vi "DFD FXP Postprocessing (I16, nCh).vi"(5 "input range":dbl=1.0, 6 "history in":i16[](array[numeric]), 7 "# channels":i32=1, 8 "error in (no error)":errorcluster, 10 "filter":T1={"mSRate_Fs"=1.0, "mSRate_Version"="2.0", "mSRate_Comments"="", "mSRate_OrgCoef"={"type"=enum."Undefined", "gain"=1.0, "coef a (k)"=[], "coef b (v)"=[]}, "mSRate_CurCoef"={"type"=enum."Undefined", "gain"=1.0, "coef a (k)"=[], "coef b (v)"=[]}, "mSRate_Quantized?"=FALSE, "mSRate_QCoef"={"type"=enum."Undefined", "gain"=1.0, "coef a (k)"=[], "coef b (v)"=[]}, "mSRate_QSettings"=[], "mSRate_Order"=0, "mSRate_Scaling"={"mSRate_ScaleByPowerOf2?"=FALSE, "mSRate_ScaleType"=enum."No Norm"}} {"mSRate_QSettings"."source" items=["Coef a/k"=0, "Coef b/v"=7, "Input"=1, "Output"=2, "Multiplicand"=3, "Product"=4, "Sum"=5, "Delay"=6, "Gain"=8]}, 11 "signal in":i16[](array[numeric]) format="%.0x") -> (0 "error out":errorcluster, 3 "signal out":dbl[][](array[numeric]), 4 "history out":i16[](array[numeric]))   [LabVIEW 2017, in "NI_DigFilterLicensed.lvlib"]
doc: "Converts the output signal of a fixed-point filter from a fixed-point integer representation to a floating-point representation. You must manually select the polymorphic instance you want to use."
uses:
  <vilib>/addons/Digital Filter Design/NI_DigFilterLicensed.lvlib
  <vilib>/addons/Digital Filter Design/_Objects.llb/DFD Filter Obj.ctl
  <vilib>/addons/Digital Filter Design/_Objects.llb/DFD Filter Coef.ctl
  <vilib>/addons/Digital Filter Design/_Objects.llb/DFD Filter Structure Type Selector.ctl
  <vilib>/addons/Digital Filter Design/_Objects.llb/dfd_Internal Quantization Settings.ctl
  <vilib>/addons/Digital Filter Design/_Objects.llb/dfd_Internal Quantization Srcs.ctl
  <vilib>/addons/Digital Filter Design/_Objects.llb/DFD Coef Norm Type.ctl
  <vilib>/addons/Digital Filter Design/NI_DigFilter_FXP.lvlib
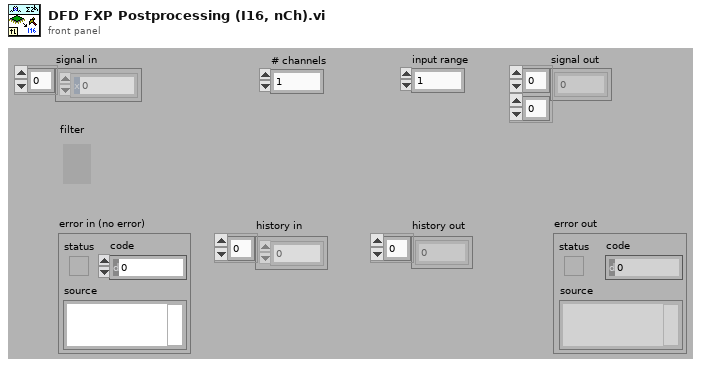
[diagram p1: front panel]
types:
  T1 = typedef "NI_DigFilterLicensed.lvlib/DFD Filter Obj.ctl" = cluster{"mSRate_Fs":dbl, "mSRate_Version":string, "mSRate_Comments":string, "mSRate_OrgCoef":T2, "mSRate_CurCoef":T2, "mSRate_Quantized?":bool, "mSRate_QCoef":T2, "mSRate_QSettings":T4[], "mSRate_Order":i32, "mSRate_Scaling":cluster{"mSRate_ScaleByPowerOf2?":bool, "mSRate_ScaleType":T6}}
  T2 = typedef "NI_DigFilterLicensed.lvlib/DFD Filter Coef.ctl" = cluster{"type":T3, "gain":dbl, "coef a (k)":dbl[], "coef b (v)":dbl[]}
  T3 = typedef "NI_DigFilterLicensed.lvlib/DFD Filter Structure Type Selector.ctl" = enum16{"Undefined", "FIR Direct Form", "FIR Direct Form Transposed", "FIR Symmetric", "FIR Antisymmetric", "IIR Direct Form I", "IIR Direct Form I Transposed", "IIR Direct Form II", "IIR Direct Form II Transposed", "IIR Cascaded Second Order Sections Form I", "IIR Cascaded Second Order Sections Form I Transposed", "IIR Cascaded Second Order Sections Form II", "IIR Cascaded Second Order Sections Form II Transposed", "Lattice Allpass (basic sections)", "Lattice Allpass (one multiplier sections)", "Lattice Allpass (normalized sections)", "Lattice AR (basic sections)", "Lattice AR (one multiplier sections)", "Lattice AR (normalized sections)", "Lattice MA (minimum phase)", "Lattice MA (maximum phase)", "Lattice ARMA (basic sections)", "Lattice ARMA (one multiplier sections)", "Lattice ARMA (normalized sections)"}
  T4 = typedef "NI_DigFilterLicensed.lvlib/dfd_Internal Quantization Settings.ctl" = cluster{"source":T5, "wl":i16, "iwl":i16, "overflow mode":enum16{"Saturation", "Wrap"}, "rounding mode":enum16{"Nearest", "Truncation"}, "signed?":bool}
  T5 = typedef "NI_DigFilterLicensed.lvlib/dfd_Internal Quantization Srcs.ctl" = u16
  T6 = typedef "NI_DigFilterLicensed.lvlib/DFD Coef Norm Type.ctl" = enum16{"No Norm", "Time Domain 1-Norm", "Time Domain 2-Norm", "Time Domain Inf-Norm"}
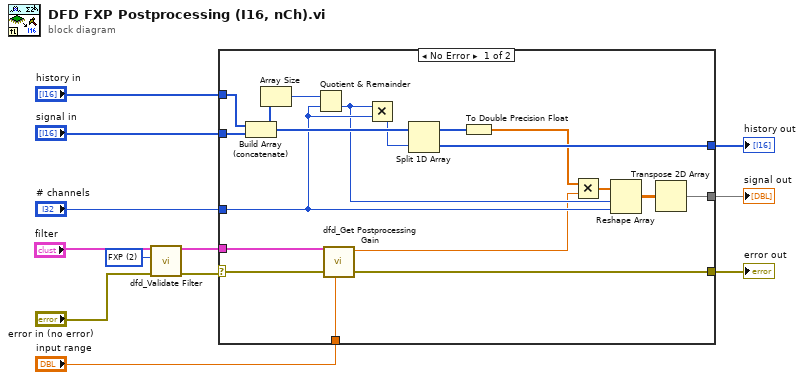
[diagram p0: block diagram]
diagram:
  w6 = u16 2 items=["Auto", "FLP Only", "FXP"] ("check option")
  n1 = call <vilib>:"dfd_Validate Filter.vi"("error in (no error)"="error in (no error)", "check option"=w6, "filter in"="filter") -> ("error out"=w3:errorcluster, "filter out"=w2:T1)  [unwired: 7 out]
  n2 = case shown="No Error" w3 {
    selector: w3 -> [w13 w30]
    tunnel: "signal in" -> [w28 _]
    tunnel: "history in" -> [w27 _]
    tunnel: [w24 _] -> w10
    tunnel: [w21 _] -> w9
    tunnel: "# channels" -> [w20 _]
    tunnel: w2 -> [w16 _]
    tunnel: [w13 w30] -> w7
    tunnel: "input range" -> [w14 _]
    frame No Error {
      n3 = Build Array (concatenate)(w27, w28) -> (w26:i16[])
      n4 = Array Size(array=w26) -> (size(s)=w29:i32)
      n5 = Quotient & Remainder(x=w29, y=w20) -> (floor(x/y)=w19:i32)  [unwired: 1 out]
      n6 = call <vilib>:"dfd_Get Postprocessing Gain.vi"("input range"=w14, "filter"=w16) -> ("integer gain"=w15:dbl)  [unwired: 9 out]
      n7 = Multiply(x=w19, y=w20) -> (x*y=w25:i32)
      n8 = Split 1D Array(array=w26, index=w25) -> (first subarray=w18:i16[], second subarray=w24:i16[])
      n9 = To Double Precision Float(number=w18) -> (double precision float=w17:dbl[])
      n10 = Multiply(x=w17, y=w15) -> (x*y=w23:dbl[])
      n11 = Reshape Array(w23, w19, w20) -> (w22:dbl[][])
      n12 = Transpose 2D Array(2D array=w22) -> (transposed array=w21:dbl[][])
    }
    frame Error {
    }
  }
  "signal out" <- w9
  "error out" <- w7
  "history out" <- w10
